vi "update arm state.vi"(10 "Bottom LS":bool, 11 "Arm state":T1=enum."Feeder") -> (3 "Arm state":T1=enum."Feeder")   [LabVIEW 2014]
doc: "Switches between arm states based on Teleop button presses.\n\nSee block diagram for specific functionality."
uses:
  Arm State.ctl
  Robot Global Data.vi
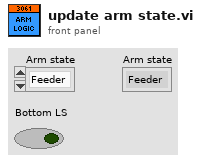
[diagram p1: front panel]
types:
  T1 = typedef "Arm State.ctl" = enum16{"Ground", "Level", "Feeder", "Vertical"}
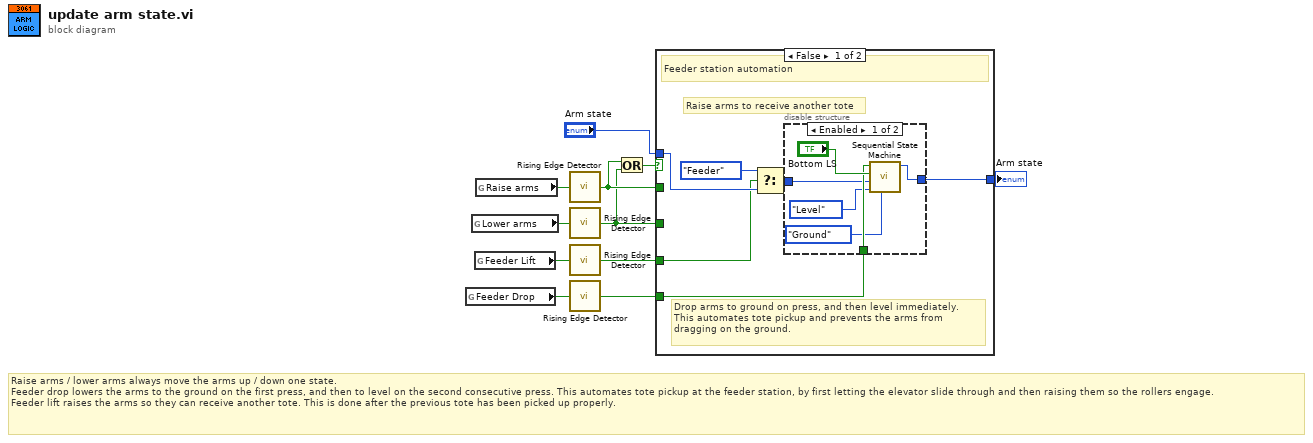
[diagram p0: block diagram]
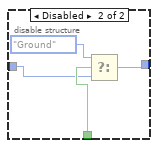
[diagram p2: hidden frame]
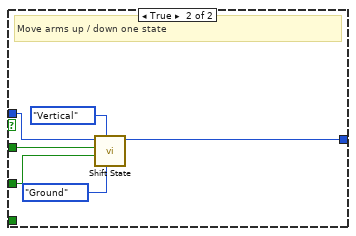
[diagram p3: hidden frame]
diagram:
  # "Raise arms / lower arms always move the arms up / down one state.\nFeeder drop lowers the arms to the ground on the first press, and then to level on the second consecutive press. This automates tote pickup at the feeder station, by first letting the elevator slide through and then raising them so the rollers engage.\nFeeder lift raises the arms so they can receive another tote. This is done after the previous tote has been picked up properly."
  n1 = global read "Robot Global Data.vi" "Feeder Drop"() -> (w9:bool)
  n2 = global read "Robot Global Data.vi" "Lower arms"() -> (w10:bool)
  n3 = global read "Robot Global Data.vi" "Feeder Lift"() -> (w8:bool)
  n4 = global read "Robot Global Data.vi" "Raise arms"() -> (w11:bool)
  n5 = call "Rising Edge Detector.vi"("Input"=w11) -> ("Rising edge?"=w6:bool)
  n6 = call "Rising Edge Detector.vi"("Input"=w10) -> ("Rising edge?"=w5:bool)
  n7 = call "Rising Edge Detector.vi"("Input"=w8) -> ("Rising edge?"=w4:bool)
  n8 = call "Rising Edge Detector.vi"("Input"=w9) -> ("Rising edge?"=w3:bool)
  n9 = Or(x=w6, y=w5) -> (x .or. y?=w7:bool)
  n10 = case shown="False" w7 {
    tunnel: w6 -> [_ w31]
    tunnel: w5 -> [_ w30]
    tunnel: [w12 w29] -> w1
    tunnel: w4 -> [w15 _]
    tunnel: w3 -> [w14 _]
    tunnel: "Arm state" -> [w17 w28]
    frame False {
      # "Raise arms to receive another tote"
      # "Drop arms to ground on press, and then level immediately.\nThis automates tote pickup and prevents the arms from\ndragging on the ground."
      # "Feeder station automation"
      n11 = Select(t=Arm_State."Feeder" ("Arm state"), s=w15, f=w17) -> (s? t:f=w13:T1)
      n12 = disable-structure shown="Enabled" {
        disable-tunnel: w14 -> [w22 w27]
        disable-tunnel: w13 -> [w21 w26]
        disable-tunnel: [w18 w24] -> w12
        frame Enabled {
          n13 = call "Sequential State Machine.vi"("Base State"=Arm_State."Ground" ("Arm state"), "Change State"=Arm_State."Level" ("Arm state"), "Old State"=w21, "Change Condition"="Bottom LS", "Button Press"=w22) -> ("Out State"=w18:i32)  [unwired: 6 in]
        }
        frame Disabled {
          n14 = Select(t=Arm_State."Ground" ("Arm state"), s=w27, f=w26) -> (s? t:f=w24:T1)
        }
      }
    }
    frame True {
      # "Move arms up / down one state"
      n15 = call "Shift State.vi"("Lower bound"=Arm_State."Ground" ("Arm state"), "Upper bound"=Arm_State."Vertical" ("Arm state"), "Decrement"=w30, "Increment"=w31, "State in"=w28) -> ("State out"=w29:i32)  [unwired: 6 in]
    }
  }
  "Arm state" <- w1
